vi "WriteReadDragPI_YCC.vi"() -> ()   [LabVIEW 2014]
panel:
  in  "Move to Position":bool
  in  "Clear one          all":bool
  in  "Clear Save Position":bool
  in  "Save Position":bool
  in  "Tab Control":enum32{"StandBy", "Drag", "Single WriteRead"}(tab)
  in  "Update ScanRate?":bool
  out "Save Position (um)":dbl[][](array[numeric])
  in  "Clear index (row)":i32
  in  "Move index (row)":i32
  in  "Velocity values":dbl[](array[numeric]) format="%.6f"
  out "XY Position":cluster{"X":dbl, "Y":dbl}[](graph)
  in  "Z  (um)":dbl=50.0 format="%.4f"
  out "Current Z (um)":dbl
  in  "Move Z?":bool
  in  "Adjust to Single Read":bool
  in  "Chang X?":bool
  in  "X Move to (um)":dbl=50.0 format="%_6g"
  in  "Chang Y?":bool
  in  "Y Move to (um)":dbl=50.0 format="%_6g"
  in  "Z Move to (um)":dbl=50.0 format="%_6g"
  in  "Chang Z?":bool
  in  "milliseconds to wait":u32=200
  out "Current Position Z (um)":dbl format="%.4f"
  out "Current Position Y (um)":dbl format="%.4f"
  out "Current Position X (um)":dbl format="%.4f"
  in  "read #":i32=1
  in  "Adjust to cursor":bool=TRUE
  in  "Update ScanRate?":bool
  out "Velocity":dbl[](array[numeric]) format="%.6f"
  in  "Move to (50,50,50) ?":bool
  in  "STOP":bool
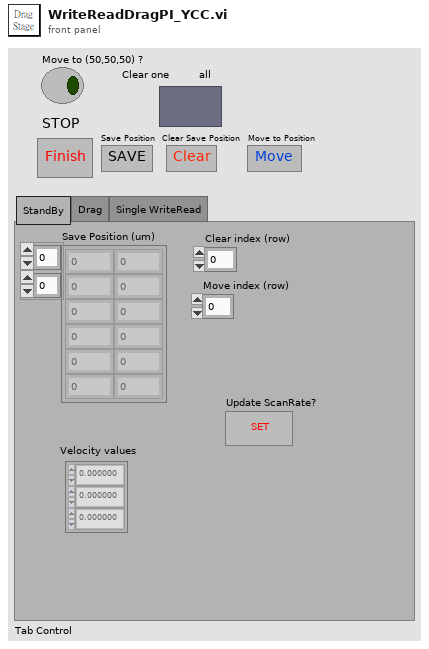
[diagram p1: front panel]
types:
  T1 = enum16{"StandBy", "Drag", "Single WriteRead", "Move to 50,50,50"}
  T2 = cluster{"Real Current Commanded position (um)":dbl, "Real Current Commanded position (um)":dbl}
  T3 = typedef "LVPointDoubleTypeDef.ctl" = cluster{"Cursor X":dbl, "Cursor Y":dbl}
  T4 = cluster{"position (um)":dbl, "position (um)":dbl}
  T5 = cluster{"Position wrote to three axis (um)":dbl, "Position wrote to three axis (um)":dbl}
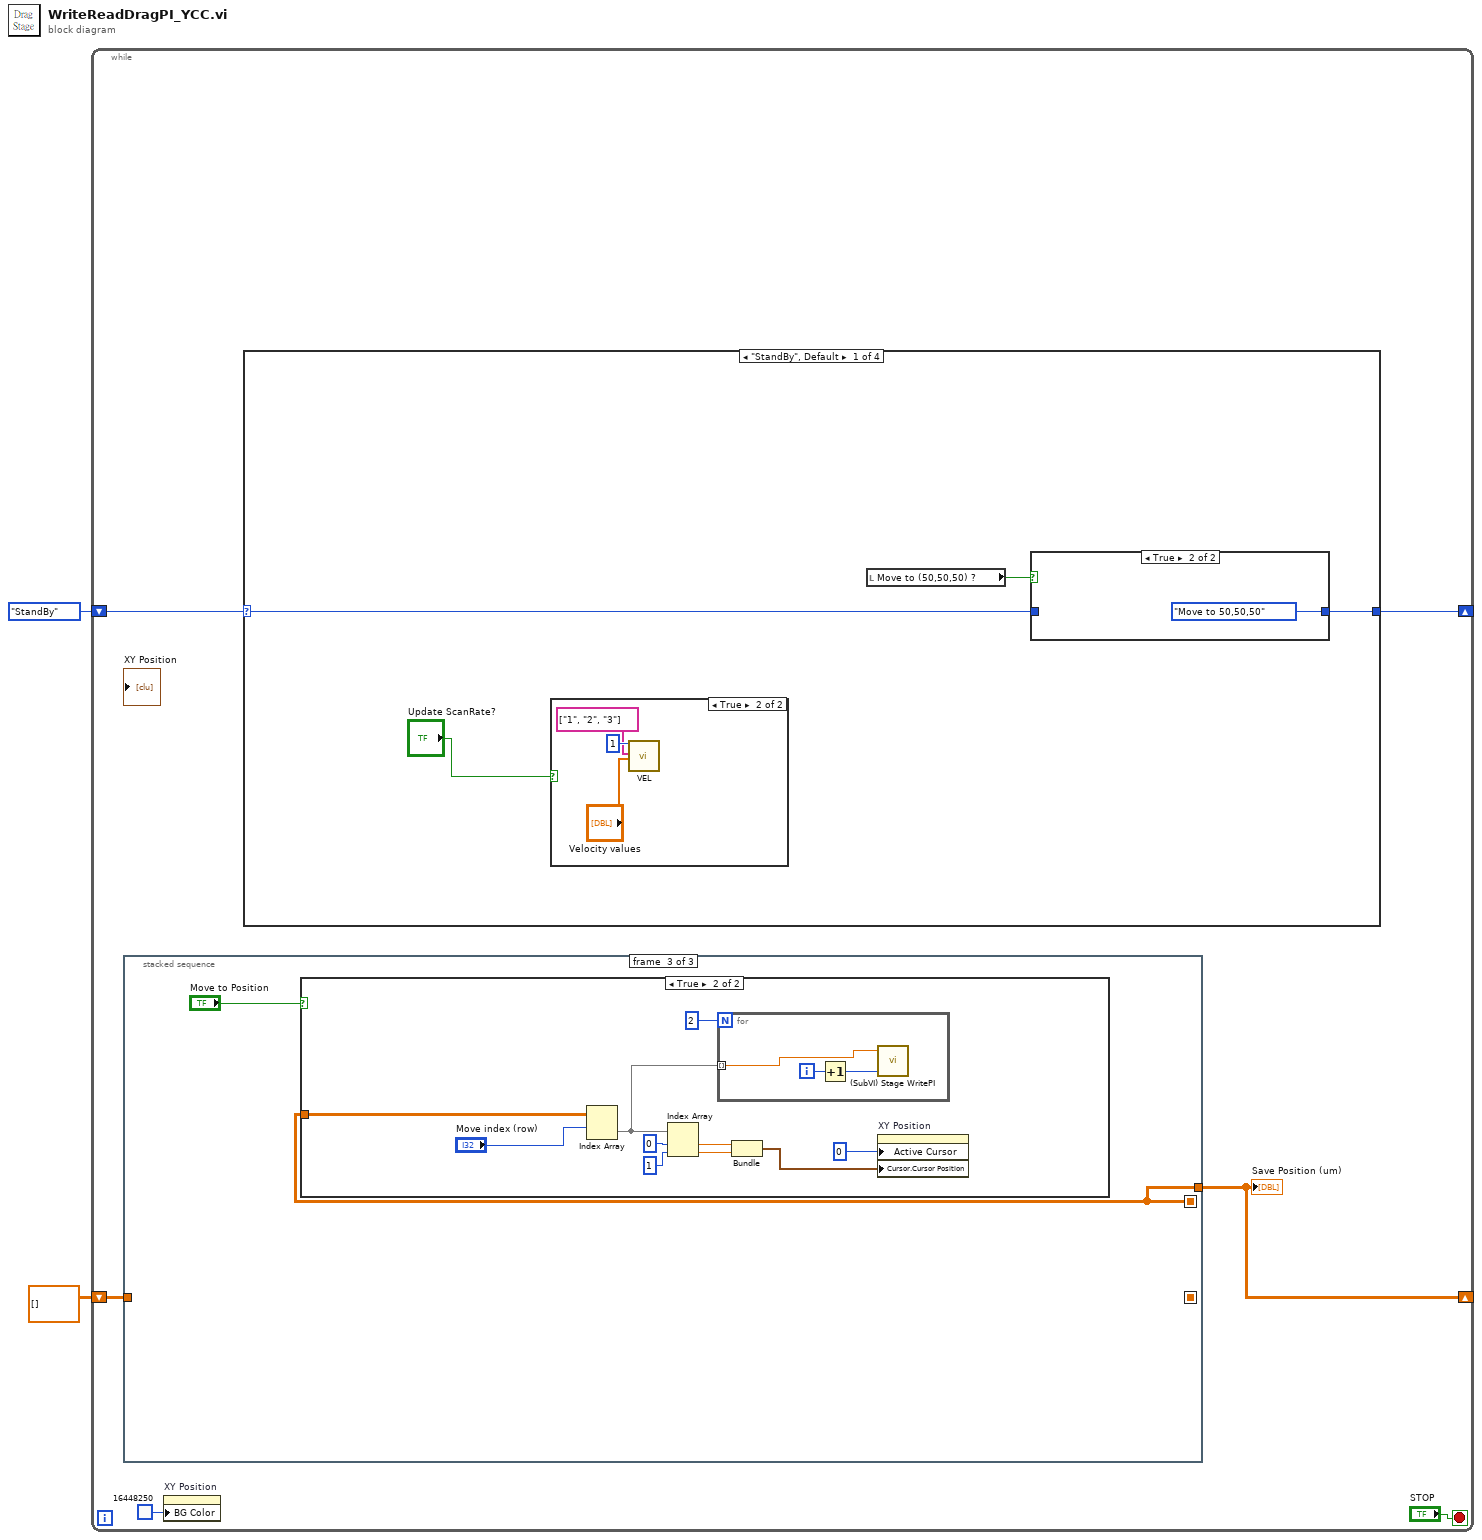
[diagram p0: block diagram]
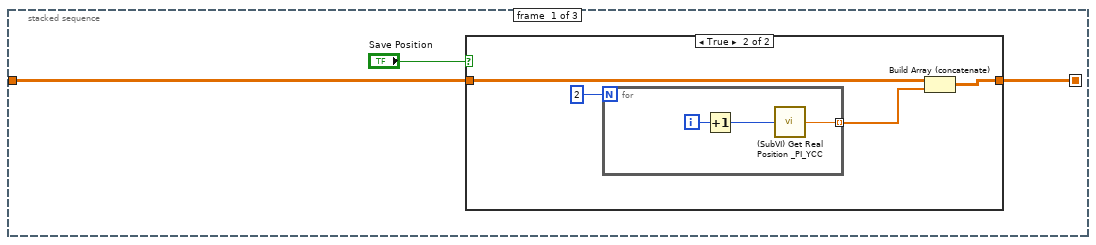
[diagram p2: hidden frame]
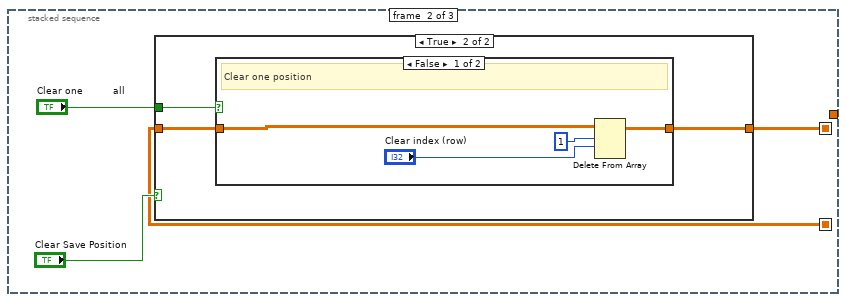
[diagram p4: hidden frame]
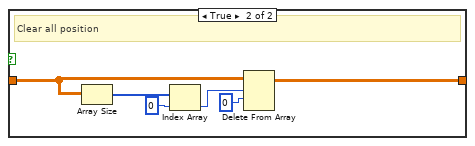
[diagram p6: hidden frame]
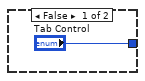
[diagram p9: hidden frame]
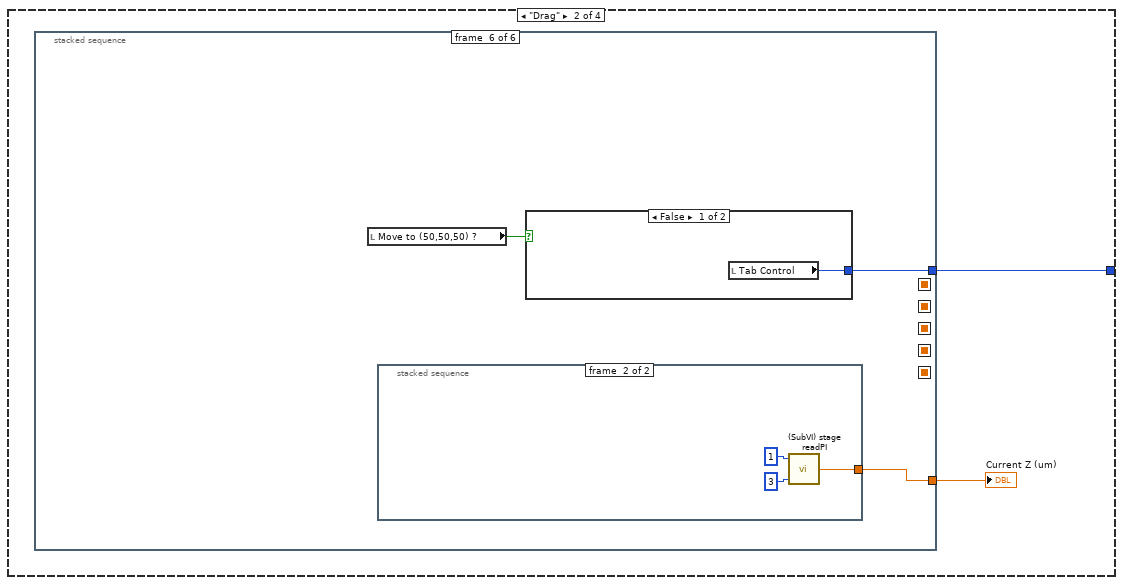
[diagram p10: hidden frame]
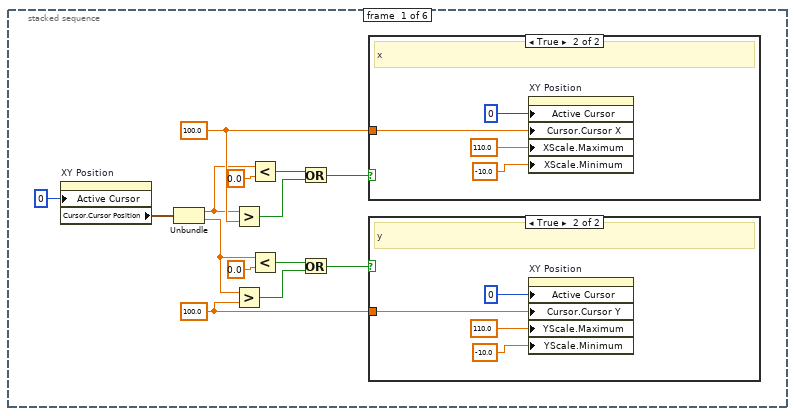
[diagram p11: hidden frame]
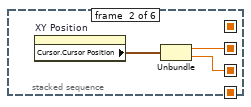
[diagram p14: hidden frame]
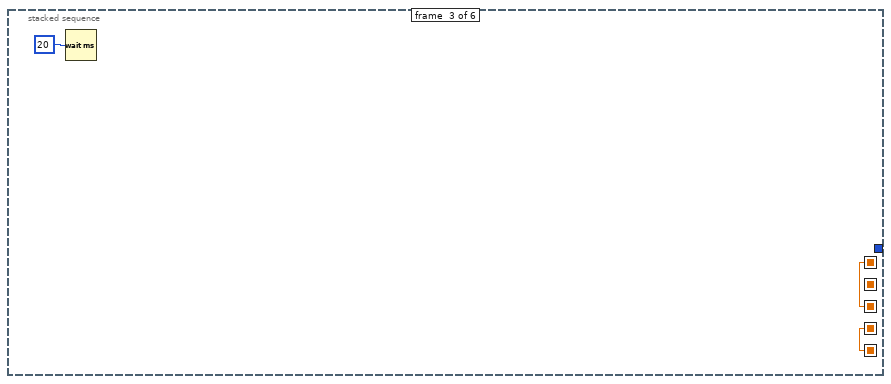
[diagram p15: hidden frame]
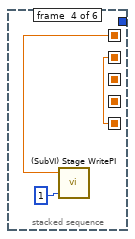
[diagram p16: hidden frame]
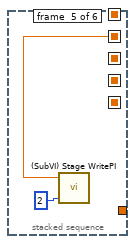
[diagram p17: hidden frame]
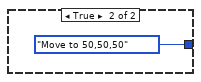
[diagram p18: hidden frame]
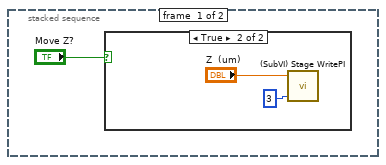
[diagram p19: hidden frame]
diagram:
  n1 = while {
    shift-right: [w8] -> _
    shift-left: T1."StandBy" ("Enum") -> [w6]
    shift-right: [w4] -> _
    shift-left: dbl[][] [] -> [w5]
    stop <- "STOP" stop-if-true
    n2 = stacked-sequence {
      seq-local: [w9 _ _] -> [_ w21 _]
      seq-local: [_ w22 _] -> [_ _ w39]
      tunnel: w5 -> [w10 _ _]
      tunnel: [_ _ w39] -> w4
      frame #0 {
        n3 = case shown="True" "Save Position" {
          tunnel: [w12 w14] -> w9
          tunnel: w10 -> [w12 w13]
          frame False {
          }
          frame True {
            n4 = for {
              N: 2 -> [_]
              tunnel: [w17] -> w15 mode=indexing
              i -> [w19]
              n5 = Increment(x=w19) -> (x+1=w18:i32)
              n6 = call "(SubVI) Get Real Position _PI_YCC.vi"("Axis"=w18) -> ("Real Current Commanded position (um)"=w17:dbl)  [unwired: 4 in]
            }
            n7 = Build Array (concatenate)(w13, w15) -> (w14:dbl[][])
          }
        }
      }
      frame #1 {
        n8 = case shown="True" "Clear Save Position" {
          tunnel: [w24 w25] -> w22
          tunnel: w21 -> [w24 w26]
          tunnel: "Clear one          all" -> [_ w27]
          frame False {
          }
          frame True {
            n9 = case shown="False" w27 {
              tunnel: w26 -> [w31 w37]
              tunnel: [w29 w32] -> w25
              frame False {
                # "Clear one position"
                n10 = Delete From Array(array=w31, length=1, index (row)="Clear index (row)") -> (array with subset deleted=w29:dbl[][])  [unwired: 1 in, 1 out]
              }
              frame True {
                # "Clear all position"
                n11 = Array Size(array=w37) -> (size(s)=w36:i32[])
                n12 = Index Array(array=w36, index=0) -> (element=w34:i32)
                n13 = Delete From Array(array=w37, length=w34, index (row)=0) -> (array with subset deleted=w32:dbl[][])  [unwired: 1 in, 1 out]
              }
            }
          }
        }
      }
      frame #2 {
        n14 = case shown="True" "Move to Position" {
          tunnel: w39 -> [_ w49]
          frame False {
          }
          frame True {
            n15 = Index Array(array=w49, index (row)="Move index (row)") -> (element=w45:dbl[])  [unwired: 1 in]
            n16 = Index Array(array=w45, index #1=0 ("index"), index #2=1 ("index")) -> (element #1=w42:dbl, element #2=w41:dbl)
            n17 = for {
              N: 2 -> [_]
              tunnel: w45 -> [w52] mode=indexing
              i -> [w51]
              n18 = Increment(x=w51) -> (x+1=w50:i32)
              n19 = call "(SubVI) Stage WritePI.vi"("axis"=w50, "position"=w52) -> ()  [unwired: 4 in]
            }
            n20 = Bundle("Real Current Commanded position (um)"=w42, "Real Current Commanded position (um)"=w41) -> (w40:T2)  [unwired: 1 in]
            n21 = property on="XY Position" class="XYGraph (strict)"("Active Cursor"=u32 0, "Cursor.Cursor Position"=w40) -> ()  [unwired: 2 in, 2 out]
          }
        }
      }
    }
    "Save Position (um)" <- w4
    n22 = property on="XY Position" class="XYGraph (strict)"("BG Color"=u32 16448250) -> ()  [unwired: 2 in, 2 out]
    n23 = case shown="\"StandBy\", Default" w6 {
      selector: w6 -> [w54 _ _ _]
      tunnel: [w55 w62 w108 w160] -> w8
      frame "StandBy", Default {
        n24 = case shown="True" "Update ScanRate?" {
          frame False {
          }
          frame True {
            n25 = call "VEL.vi"("System no."=1, "Axes to set"=string[] ["1", "2", "3"], "Velocity values"="Velocity values") -> ()  [unwired: 15 in, 2 out]
          }
        }
        n26 = local read "Move to (50,50,50) ?"() -> (w56:bool)
        n27 = case shown="True" w56 {
          tunnel: ["Tab Control" T1."Move to 50,50,50" ("Enum")] -> w55
          tunnel: w54 -> [_ _]
          frame False {
          }
          frame True {
          }
        }
      }
      frame "Drag" {
        n28 = stacked-sequence {
          seq-local: [_ w86 _ _ _ _] -> [_ _ w90 _ _ _]
          seq-local: [_ w87 _ _ _ _] -> [_ _ w89 _ _ _]
          seq-local: [_ _ w90 _ _ _] -> [_ _ _ w92 _ _]
          seq-local: [_ _ w89 _ _ _] -> [_ _ _ w93 _ _]
          seq-local: [_ _ _ w92 _ _] -> [_ _ _ _ w95 _]
          tunnel: [_ _ _ _ _ w99] -> w63
          tunnel: [_ _ _ _ _ w97] -> w62
          frame #0 {
            w75 = 100.0 ("y")
            w76 = 100.0 ("y")
            n29 = property on="XY Position" class="XYGraph (strict)"("Active Cursor"=u32 0) -> ("Cursor.Cursor Position"=w77:T3)  [unwired: 2 in, 2 out]
            n30 = Unbundle(w77) -> ("Cursor X"=w73:dbl, "Cursor Y"=w70:dbl)
            n31 = Greater?(x=w73, y=w76) -> (0:w68:bool)
            n32 = Greater?(x=w70, y=w75) -> (0:w65:bool)
            n33 = Less?(x=w73, y=0.0) -> (x < y?=w69:bool)
            n34 = Less?(x=w70, y=0.0) -> (x < y?=w66:bool)
            n35 = Or(x=w69, y=w68) -> (x .or. y?=w67:bool)
            n36 = Or(x=w66, y=w65) -> (x .or. y?=w64:bool)
            n37 = case shown="True" w67 {
              tunnel: w76 -> [_ w85]
              frame False {
              }
              frame True {
                # "x"
                n38 = property on="XY Position" class="XYGraph (strict)"("Active Cursor"=u32 0, "Cursor.Cursor X"=w85, "XScale.Maximum"=110.0 ("X Scale.Range:Maximum"), "XScale.Minimum"=-10.0 ("X Scale.Range:Minimum")) -> ()  [unwired: 2 in, 2 out]
              }
            }
            n39 = case shown="True" w64 {
              tunnel: w75 -> [_ w81]
              frame False {
              }
              frame True {
                # "y"
                n40 = property on="XY Position" class="XYGraph (strict)"("Active Cursor"=u32 0, "Cursor.Cursor Y"=w81, "YScale.Maximum"=110.0 ("X Scale.Range:Maximum"), "YScale.Minimum"=-10.0 ("X Scale.Range:Minimum")) -> ()  [unwired: 2 in, 2 out]
              }
            }
          }
          frame #1 {
            n41 = property on="XY Position" class="XYGraph (strict)"() -> ("Cursor.Cursor Position"=w88:T3)  [unwired: 2 in, 2 out]
            n42 = Unbundle(w88) -> ("Cursor X"=w87:dbl, "Cursor Y"=w86:dbl)
          }
          frame #2 {
            n43 = Wait (ms)(milliseconds to wait=u32 20) -> ()  [unwired: 1 out]
          }
          frame #3 {
            n44 = call "(SubVI) Stage WritePI.vi"("axis"=u32 1, "position"=w93) -> ()  [unwired: 4 in]
          }
          frame #4 {
            n45 = call "(SubVI) Stage WritePI.vi"("axis"=u32 2, "position"=w95) -> ()  [unwired: 4 in]
          }
          frame #5 {
            n46 = local read "Move to (50,50,50) ?"() -> (w98:bool)
            n47 = stacked-sequence {
              tunnel: [_ w105] -> w99
              frame #0 {
                n48 = case shown="True" "Move Z?" {
                  frame False {
                  }
                  frame True {
                    n49 = call "(SubVI) Stage WritePI.vi"("axis"=u32 3, "position"="Z  (um)") -> ()  [unwired: 4 in]
                  }
                }
              }
              frame #1 {
                n50 = call "(SubVI) stage readPI.vi"("Axis"=u32 3 ("axis"), "read #"=1) -> ("position (um)"=w105:dbl)  [unwired: 3 in]
              }
            }
            n51 = case shown="False" w98 {
              tunnel: [w100 T1."Move to 50,50,50" ("Enum")] -> w97
              frame False {
                n52 = local read "Tab Control"() -> (w100:enum32{"StandBy", "Drag", "Single WriteRead"})
              }
              frame True {
              }
            }
          }
        }
        "Current Z (um)" <- w63
      }
      frame "Single WriteRead" {
        n53 = stacked-sequence {
          seq-local: [_ _ _ _ w120 _ _ _ _] -> [_ _ _ _ _ w134 _ _ _]
          seq-local: [_ _ _ _ w119 _ _ _ _] -> [_ _ _ _ _ w133 _ _ _]
          seq-local: [_ _ _ _ _ w134 _ _ _] -> [_ _ _ _ _ _ w138 _ _]
          seq-local: [_ _ _ _ _ w133 _ _ _] -> [_ _ _ _ _ _ w137 _ _]
          tunnel: [_ _ _ _ _ w131 _ _ _] -> w108
          frame #0 {
            # "write x"
            n54 = case shown="True" "Chang X?" {
              frame False {
              }
              frame True {
                n55 = call "(SubVI) Stage WritePI.vi"("axis"=u32 1, "position"="X Move to (um)") -> ()  [unwired: 4 in]
              }
            }
          }
          frame #1 {
            # "write y"
            n56 = case shown="True" "Chang Y?" {
              frame False {
              }
              frame True {
                n57 = call "(SubVI) Stage WritePI.vi"("axis"=u32 2, "position"="Y Move to (um)") -> ()  [unwired: 4 in]
              }
            }
          }
          frame #2 {
            n58 = case shown="True" "Chang Z?" {
              frame False {
              }
              frame True {
                n59 = call "(SubVI) Stage WritePI.vi"("axis"=u32 3, "position"="Z Move to (um)") -> ()  [unwired: 4 in]
              }
            }
          }
          frame #3 {
            n60 = Wait (ms)(milliseconds to wait="milliseconds to wait") -> ()  [unwired: 1 out]
          }
          frame #4 {
            n61 = for {
              N: 3 -> [_]
              tunnel: [w127] -> w125 mode=indexing
              i -> [w130]
              n62 = Increment(x=w130) -> (x+1=w129:i32)
              n63 = call "(SubVI) stage readPI.vi"("Axis"=w129, "read #"="read #") -> ("position (um)"=w127:dbl)  [unwired: 3 in]
            }
            n64 = Index Array(array=w125, index #1=0 ("index"), index #2=1 ("index"), index #3=2 ("index")) -> (element #1=w120:dbl, element #2=w119:dbl, element #3=→"Current Position Z (um)":dbl)
            "Current Position X (um)" <- w120
            "Current Position Y (um)" <- w119
          }
          frame #5 {
            n65 = local read "Move to (50,50,50) ?"() -> (w132:bool)
            n66 = case shown="True" w132 {
              tunnel: [w135 T1."Move to 50,50,50" ("Enum")] -> w131
              frame False {
                n67 = local read "Tab Control"() -> (w135:enum32{"StandBy", "Drag", "Single WriteRead"})
              }
              frame True {
              }
            }
          }
          frame #6 {
            n68 = case shown="True" "Adjust to cursor" {
              tunnel: w138 -> [_ w141]
              tunnel: w137 -> [_ w140]
              frame False {
              }
              frame True {
                n69 = Bundle("position (um)"=w141, "position (um)"=w140) -> (w142:T4)  [unwired: 1 in]
                n70 = property on="XY Position" class="XYGraph (strict)"("Cursor.Cursor Position"=w142) -> ()  [unwired: 2 in, 2 out]
              }
            }
          }
          frame #7 {
            n71 = case shown="True" "Adjust to Single Read" {
              frame False {
              }
              frame True {
                n72 = stacked-sequence {
                  seq-local: [w144 _] -> [_ w155]
                  frame #0 {
                    n73 = for {
                      N: 3 -> [_]
                      tunnel: [w146] -> w144 mode=indexing
                      i -> [w148]
                      n74 = Increment(x=w148) -> (x+1=w147:i32)
                      n75 = call "(SubVI) Get Real Position _PI_YCC.vi"("Axis"=w147) -> ("Real Current Commanded position (um)"=w146:dbl)  [unwired: 4 in]
                    }
                  }
                  frame #1 {
                    n76 = Index Array(array=w155, index #1=0 ("index"), index #2=1 ("index"), index #3=2 ("index")) -> (element #1=w151:dbl, element #2=w150:dbl, element #3=w149:dbl)
                    n77 = local write "X Move to (um)"(w151) -> ()
                    n78 = local write "Y Move to (um)"(w150) -> ()
                    n79 = local write "Z Move to (um)"(w149) -> ()
                  }
                }
              }
            }
          }
          frame #8 {
            n80 = case shown="True" "Update ScanRate?" {
              frame False {
              }
              frame True {
                n81 = call "VEL?.vi"("System no."=1, "All axes?"=TRUE) -> ("Velocity"=→"Velocity":dbl[])  [unwired: 16 in, 1 out]
              }
            }
          }
        }
      }
      frame "Move to 50,50,50" {
        w160 = T1."StandBy" ("Enum")
        n82 = case shown="True" "Move to (50,50,50) ?" {
          frame False {
          }
          frame True {
            n83 = stacked-sequence {
              seq-local: [w162 _] -> [_ w163]
              frame #0 {
                w162 = 50.0 ("Position wrote to three axis (um)")
                n84 = call "(SubVI) Write to Three AxisesPI_YCC.vi"("Position wrote to three axis (um)"=w162) -> ()  [unwired: 4 in]
              }
              frame #1 {
                n85 = Bundle("Position wrote to three axis (um)"=w163, "Position wrote to three axis (um)"=w163) -> (w164:T5)  [unwired: 1 in]
                n86 = property on="XY Position" class="XYGraph (strict)"("Cursor.Cursor Position"=w164) -> ()  [unwired: 2 in, 2 out]
              }
            }
          }
        }
        n87 = local write "Tab Control"(w160) -> ()
      }
    }
  }
